vi "BuildTestFromProjectItem_LibraryWithTheory_BuildsTestSuiteWithTheory.vi"() -> ()   [LabVIEW 2017, in "LVUnitTestBuilder.Tests.lvlib"]
uses:
  LVUnitTestBuilder.Tests.lvlib
  LVUnitTestBuilder/LVUnitTestBuilder.lvclass
  TestSuite/TestSuite.lvclass
  Theory/Theory.lvclass
  TestSuite/TestSuite.lvclass/TestSuite.ctl
  TestSuite/ReadTests.vi
  Test/Test.lvclass
  Assertion/Assertion.lvlib
panel:
  out "error out":errorcluster
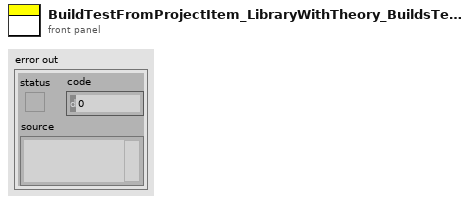
[diagram p1: front panel]
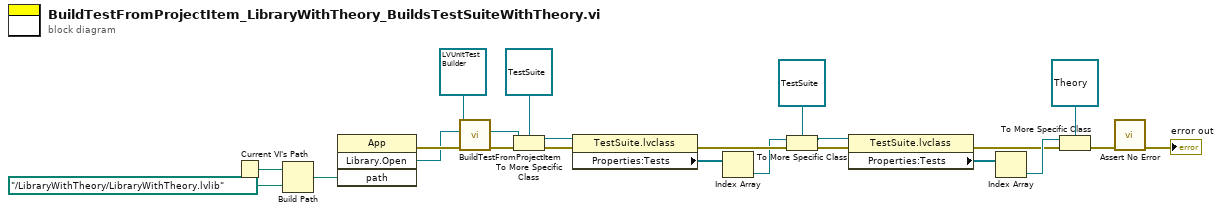
[diagram p0: block diagram]
diagram:
  n1 = Current VI's Path() -> (path=w16:path)
  n2 = Build Path(base path=w16, name or relative path=path "../LibraryWithTheory/LibraryWithTheory.lvlib") -> (appended path=w15:path)
  n3 = invoke class="App" method="Library.Open"("path"=w15) -> (error out=w19:errorcluster, "Open Library"=w18:refnum<vi>)  [unwired: 3 in, 2 out]
  n4 = call-dynamic "BuildTestFromProjectItem.vi"("error in (no error)"=w19, "ProjectItem Refnum"=w18, "LVUnitTestBuilder in"=refnum<class "LVUnitTestBuilder.lvclass"> refnum ("LVUnitTestBuilder")) -> ("error out"=w20:errorcluster, "Test"=w22:refnum<class "Test.lvclass">)  [unwired: 6 in, 1 out]
  n5 = To More Specific Class(target class=refnum<class "TestSuite.lvclass"> refnum ("TestSuite.lvclass"), reference=w22, error in=w20) -> (specific class reference=w13:refnum<class "TestSuite.lvclass">, error out=w14:errorcluster)
  n6 = property class="TestSuite.lvclass"(reference=w13, error in=w14) -> (error out=w11:errorcluster, "Properties:Tests"=w12:refnum<class "Test.lvclass">[])  [unwired: 1 out]
  n7 = Index Array(array=w12) -> (element=w10:refnum<class "Test.lvclass">)  [unwired: 1 in]
  n8 = To More Specific Class(target class=refnum<class "TestSuite.lvclass"> refnum ("TestSuite.lvclass"), reference=w10, error in=w11) -> (specific class reference=w1:refnum<class "TestSuite.lvclass">, error out=w7:errorcluster)
  n9 = property class="TestSuite.lvclass"(reference=w1, error in=w7) -> (error out=w3:errorcluster, "Properties:Tests"=w2:refnum<class "Test.lvclass">[])  [unwired: 1 out]
  n10 = Index Array(array=w2) -> (element=w5:refnum<class "Test.lvclass">)  [unwired: 1 in]
  n11 = To More Specific Class(target class=refnum<class "Theory.lvclass"> refnum ("TestCase.lvlib:Theory.lvclass"), reference=w5, error in=w3) -> (error out=w4:errorcluster)  [unwired: 1 out]
  n12 = call "Assert No Error.vi"("error in (no error)"=w4) -> ("error out"=→"error out":errorcluster)  [unwired: 10 in]
